vi "Event-Snapshot.vi"(8 "error in (no error)":errorcluster, 10 "Data ref. in":refnum<data-value>, 11 "UI ref. in":refnum<data-value>) -> (0 "error out":errorcluster, 2 "Data ref.":refnum<data-value>, 3 "UI ref.":refnum<data-value>)   [LabVIEW 2013, in "CameraVision.lvlib" / "CV-UI.lvclass"]
uses:
  CV-UI.lvclass
  Main/CV-Main.lvclass
  Control-names.ctl
  Main/CV-Main.lvclass/CV-Main.ctl
  Main/Acquisition/CV-Acquisition.lvclass/CV-Acquisition.ctl
  CV-UI.lvclass/CV-UI.ctl
  Main/Read Acquis params.vi
  Main/Acquisition/Read Manual trigger ID.vi
  Read Control refs.vi
  Main/Acquisition/CV-Acquisition.lvclass
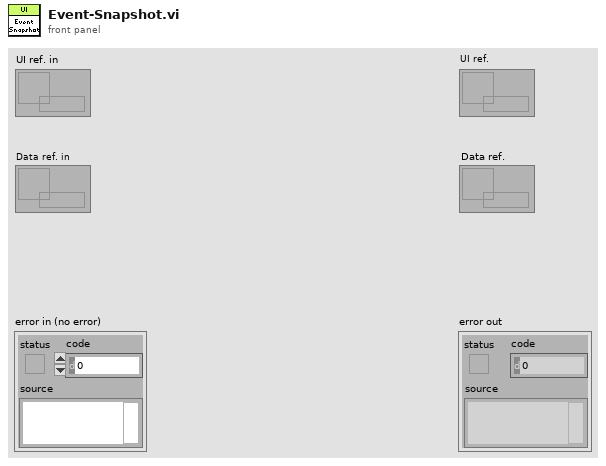
[diagram p1: front panel]
types:
  T1 = typedef "CameraVision.lvlib/CV-UI.lvclass/Control-names.ctl" = enum16{"Start acquisition", "Activate", "Stop acquisition", "Settings type", "Load settings", "Save settings", "Import images", "Camera selector", "Image type selector", "Batch browser", "Image refresh", "Parameter tabs", "Displays", "Processing tabs", "Processing selector", "Map characteristic", "Show info", "Manual trigger"}
  T2 = enum8{"Enabled", "Disabled", "Disabled and Grayed Out"}
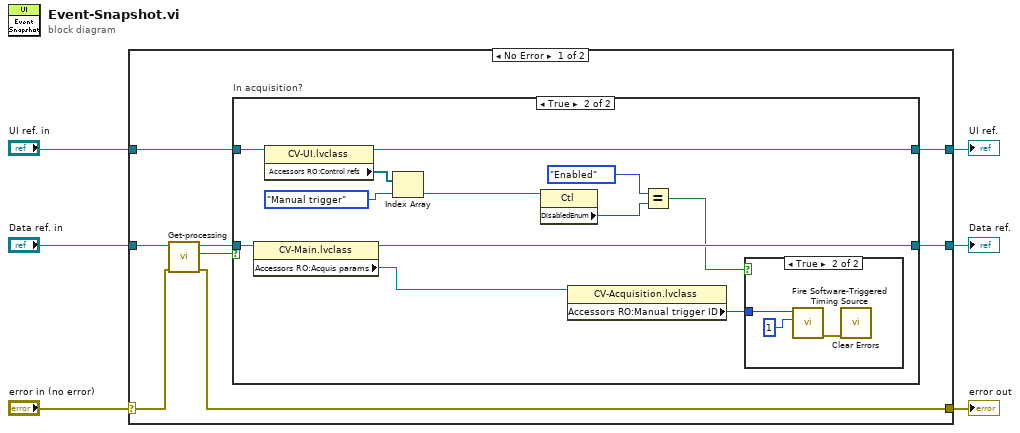
[diagram p0: block diagram]
diagram:
  n1 = case shown="No Error" "error in (no error)" {
    selector: "error in (no error)" -> [w8 w34]
    tunnel: [w7 w34] -> w5
    tunnel: [w11 w33] -> w3
    tunnel: "UI ref. in" -> [w9 w33]
    tunnel: "Data ref. in" -> [w14 w32]
    tunnel: [w10 w32] -> w1
    frame No Error {
      n2 = call "Get-processing.vi"("error in (no error)"=w8, "Data ref. in"=w14) -> ("error out"=w7:errorcluster, "Processing?"=w12:bool, "Data ref."=w13:refnum<data-value>)  [unwired: 7 in]
      n3 = case "In acquisition?" shown="True" w12 {
        tunnel: w9 -> [w16 w25]
        tunnel: w13 -> [w15 w28]
        tunnel: [w16 w22] -> w11
        tunnel: [w15 w27] -> w10
        frame False {
        }
        frame True {
          n4 = property class="CV-Main.lvclass"(reference=w28) -> (reference out=w27:refnum<data-value>, "Accessors RO:Acquis params"=w20:refnum<data-value>)  [unwired: 1 in, 1 out]
          n5 = property class="CV-UI.lvclass"(reference=w25) -> (reference out=w22:refnum<data-value>, "Accessors RO:Control refs"=w19:refnum<vi>[])  [unwired: 1 in, 1 out]
          n6 = Index Array(array=w19, index=Control-names."Manual trigger" ("Control")) -> (element=w17:refnum<vi>)
          n7 = property class="Ctl"(reference=w17) -> ("DisabledEnum"=w24:T2)  [unwired: 1 in, 2 out]
          n8 = property class="CV-Acquisition.lvclass"(reference=w20) -> ("Accessors RO:Manual trigger ID"=w26:u8)  [unwired: 1 in, 2 out]
          n9 = Equal?(x=T2."Enabled" ("y"), y=w24) -> (x = y?=w21:bool)
          n10 = case shown="True" w21 {
            tunnel: w26 -> [_ w29]
            frame False {
            }
            frame True {
              n11 = call <vilib>:"Fire Software-Triggered Timing Source.vi"("number of ticks"=u32 1, "trigger ID"=w29) -> ("error out"=w30:errorcluster)  [unwired: 8 in, 1 out]
              n12 = call <vilib>:"Clear Errors.vi"("error in (no error)"=w30) -> ()  [unwired: 6 in, 1 out]
            }
          }
        }
      }
    }
    frame Error {
    }
  }
  "error out" <- w5
  "Data ref." <- w1
  "UI ref." <- w3
